vi "ICRA2024测试椭圆分裂0904有PID控制.vi"() -> ()   [LabVIEW 2018]
doc: "Demonstrates the use of the Network Streams functions to send LED status to the myRIO target."
uses:
  <vilib>/ErrorRing/Error Ring.xnode
  <vilib>/vision/NI_Vision_Development_Module.lvlib
panel:
  out "Image 8":T1(plugin-control)
  out "控制量ratio":dbl
  in  "拉伸的增益":dbl
  in  "收缩的增益":dbl
  in  "predefined control":dbl
  out "实际的ratio":dbl
  out "期望的ratio":dbl
  out "Swarm面积":sgl
  in  "期望长度":dbl
  in  "磁场开关":bool=TRUE
  out "数据总":dbl[][](array[numeric])
  out "pitch angle2":dbl[](array[numeric])
  out "pitch angle1":sgl[](array[numeric])
  out "direction angle":sgl[](array[numeric])
  out "磁场ratio":sgl[](array[numeric])
  out "磁场频率":sgl[](array[numeric])
  out "T":i32[](array[numeric])
  out "ratio":dbl[](array[numeric])
  out "长度1":i32[](array[numeric])
  out "长度2":i32[](array[numeric])
  in  "数据记录":bool
  out "长度1":i32
  out "长度2":i32
  out "Y Bottom":i32
  out "X Right":i32
  out "Y Top":i32
  out "X Left":i32
  in  "Rectangle 3":T2={"Left"=500, "Top"=800, "Right"=800, "Bottom"=1100}
  in  "Rectangle 2":T2={"Left"=500, "Top"=500, "Right"=800, "Bottom"=600}
  in  "Rectangle":T2={"Left"=500, "Top"=0, "Right"=800, "Bottom"=300}
  in  "Search Rect (entire image)":T3={"Left"=200, "Top"=120, "Right"=2000, "Bottom"=1920, "Rotation"=0.0} {"Rotation" format="%.2f"; "Left" scale=0.0..1024.0; "Right" scale=0.0..1024.0}
  out "备用的椭圆角度":sgl
  in  "Number of Erosion":i32=10
  in  "椭圆磁场开关":bool=TRUE
  out "Image 7":T1(plugin-control)
  in  "Acquisition Control::Acquisition Frame Rate":dbl=19.50304412841797 min=1.4211589097976685 max=44.94382095336914
  out "Stopped":bool
  in  "Stop (F) 2":bool caption="Stop (F)"
  out "Objects 2":T4(array[cluster]) {"Aspect Ratio" format="%.2f"; "Orientation" format="%.2f"; "Area" format="%.2f"; "Object Center"."Y" format="%.2f"; "Object Center"."X" format="%.2f"}
  in  "Settings 2":T5={"Objects"=0, "Threshold"=128, "Reject Border"=FALSE, "Fill Holes"=FALSE, "Min Object Size"=TRUE, "Min Size"=20000, "Max Object Size"=FALSE, "Max Size"=100, "Show Search Area"=FALSE, "Show Center"=TRUE, "Show Bounding Box"=TRUE} {"Objects" items=["Bright Objects", "Dark Objects"]; "Threshold" min=1 max=999999999 step=1; "Max Size" min=1 max=999999999 step=1; "Min Size" min=1 max=999999999 step=1}
  in  "Range 2":cluster{"Lower value":sgl, "Upper value":sgl}={"Lower value"=0.0, "Upper value"=230.0} {"Upper value" format="%.2f"; "Lower value" format="%.2f"}
  in  "Pause":bool
  out "Array":dbl[](array[numeric])
  in  "Parameter Settings":T6(tab)=enum."Ribbon Oscillating Field" caption="Field Types"
  in  "fg":dbl
  in  "pg":dbl
  in  "dg":dbl
  in  "Ag":dbl
  in  "AoOF":dbl
  in  "fo":sgl
  in  "do":sgl
  in  "oo":sgl
  in  "po":sgl
  in  "cc":sgl
  in  "pc":sgl
  in  "wc":sgl
  in  "dc":sgl
  in  "Ac":dbl
  in  "pr":sgl
  in  "Ar":dbl=8.0
  in  "wr":sgl=18.0
  in  "dr":sgl
  in  "Dis phase step":dbl
  in  "Dis phase frequency (Hz)":dbl
  in  "Dis tumbling frequency (Hz)":dbl
  in  "Dis strength(mT)":dbl
  in  "Swa strength (mT)":dbl
  in  "Swa frequency (Hz)":dbl
  in  "Swa pitch angle (deg)":dbl
  in  "Swa direction angle (deg)":dbl
  in  "Swa ratio":dbl=1.0
  in  "Pitch Angle (rotating around Constant, deg)":dbl
  in  "Ratio (A/C)":sgl=3.0
  in  "Direction Angle (deg)":sgl=90.0
  in  "Pitch Angle (rotating around Origin, deg)":sgl
  in  "Frequency (Hz)":sgl=6.0
  in  "Strength (mT)":dbl=3.0
  in  "Ar 2":dbl=5.0 caption="Ar"
  in  "ratio":sgl=1.0
  in  "运动方向":sgl
  in  "长轴方向":sgl
  in  "wr  2":sgl=8.0
  in  "速度大小":sgl
  out "时间":i32
  out "Numeric 5":i32
  in  "Stop":bool
  out "error out":errorcluster
  in  "Target IP Address":string="172.22.11.2"
  # "Overview: Magnetic field calculation, and send parameters to myRIO\nInstructions:\n1. Verify the value of Target IP Address. Set Visa resource name.\n2. Ensure RT Main.vi is already running. \n3. Run this VI. Set parameters of magnetic field."
  # "Strength (mT)"
  # "Pitch Angle (deg)"
  # "Direction Angle (deg)"
  # "Frequency (Hz)"
  # "Strength (mT)"
  # "Oscilation Frequency (Hz)"
  # "Oscilation Angle (deg)"
  # "Pitch Angle (deg)"
  # "Direction Angle (deg)"
  # "Strength (mT)"
  # "Frequency (Hz)"
  # "Pitch Angle (deg)"
  # "Direction Angle (deg)"
  # "Conical Angle (deg)"
  # "Strength (mT)"
  # "Frequency (Hz)"
  # "Pitch Angle (deg)"
  # "Direction Angle (deg)"
  # "Strength (mT)"
  # "Tumbling Frequency (Hz)"
  # "Phase Frequency (Hz)"
  # "Phase Step"
  # "Strength (mT)"
  # "Frequency (Hz)"
  # "Pitch Angle (deg)"
  # "Direction Angle (deg)"
  # "Ratio"
  # "Strength (mT)"
  # "Frequency (Hz)"
  # "Ratio (A/C)"
  # "Direction Angle (deg)"
  # "Pitch Angle (rotating around Origin, deg)"
  # "Pitch Angle (rotating around Constant, deg)"
  # "Strength (mT)"
  # "Frequency (Hz)"
  # "Pitch Angle  (deg)"
  # "longaxis"
  # "Direction Angle (deg)"
  # "ratio (l/s)"
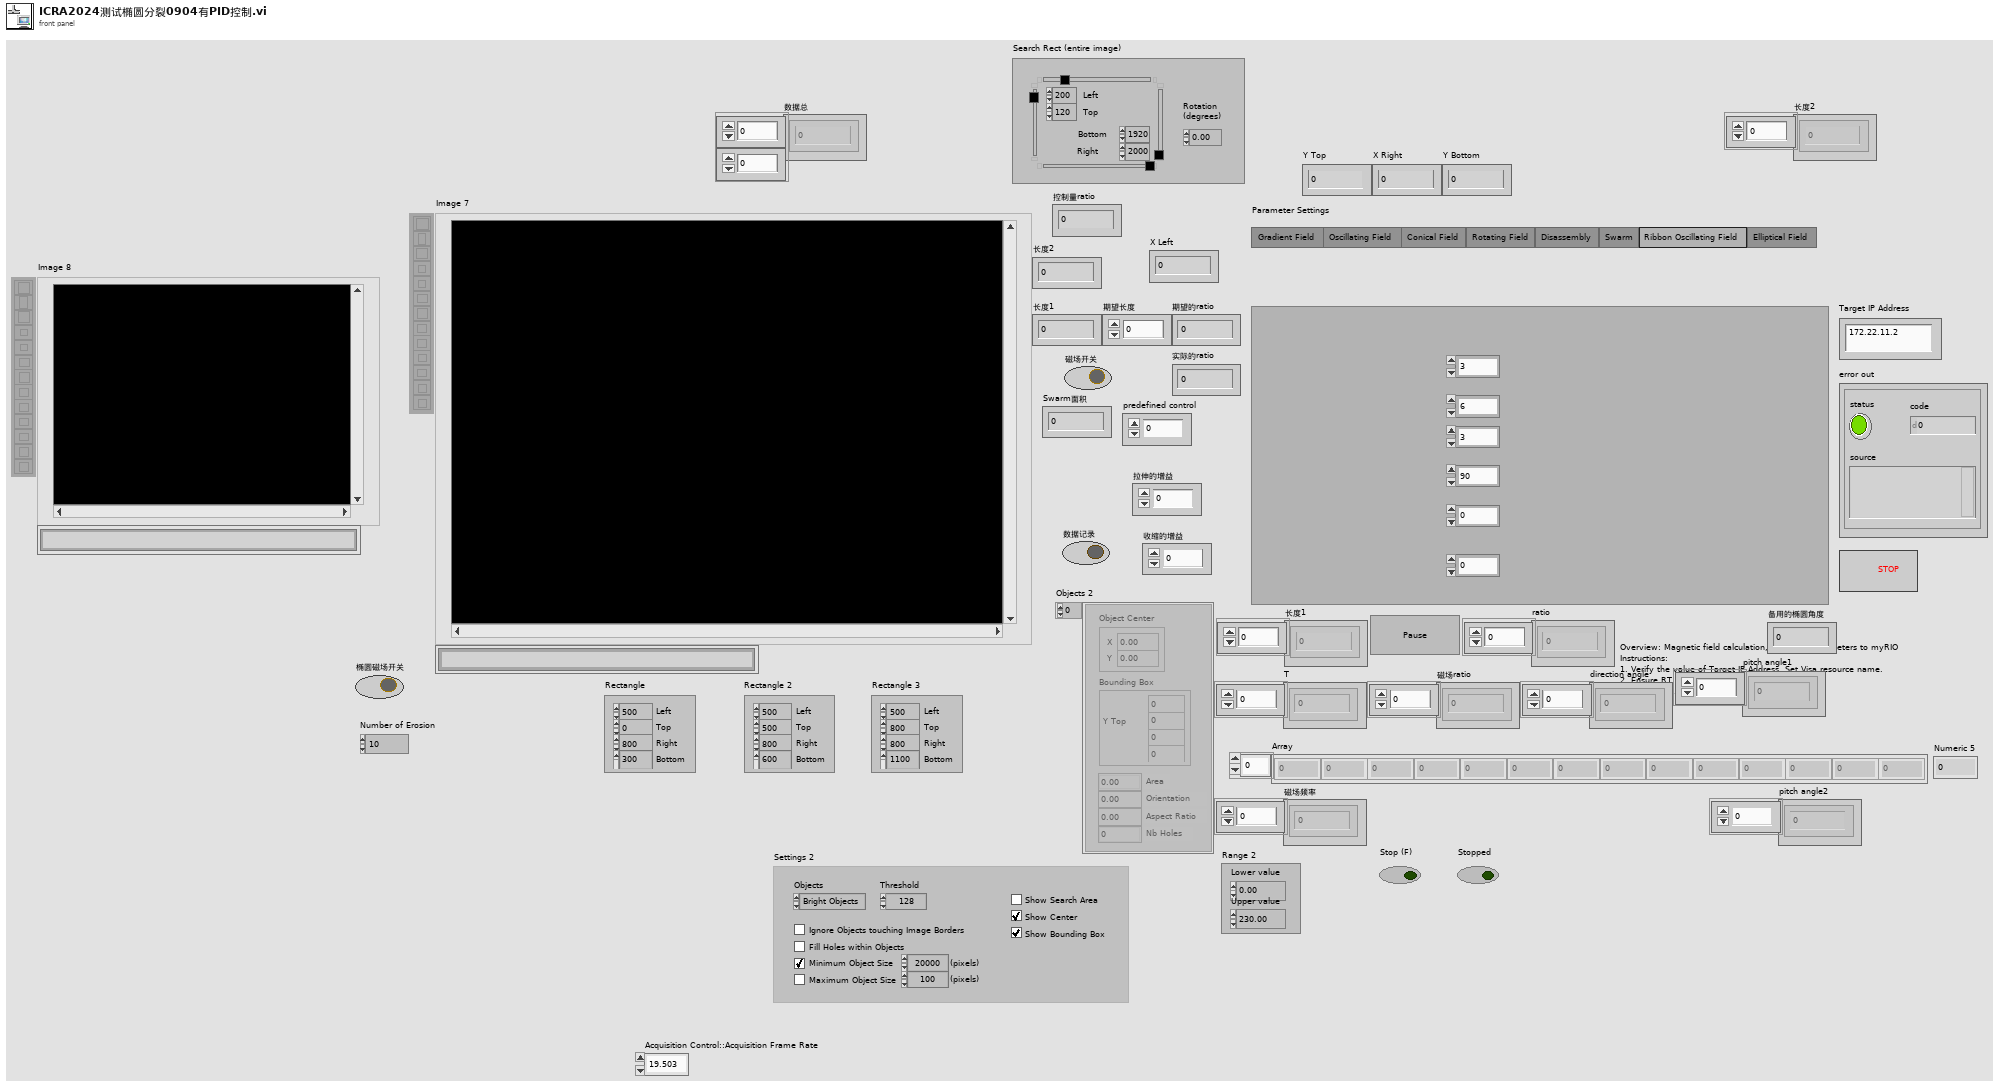
[diagram p1: front panel]
types:
  T1 = typedef "IMAQ Image.ctl" = refnum<image>
  T2 = cluster{"Left":i32, "Top":i32, "Right":i32, "Bottom":i32}
  T3 = typedef "IMAQ Rectangle" = cluster{"Left":i32, "Top":i32, "Right":i32, "Bottom":i32, "Rotation":dbl}
  T4 = cluster{"Object Center":cluster{"X":sgl, "Y":sgl}, "Bounding Box":cluster{"X Left":i32, "Y Top":i32, "X Right":i32, "Y Bottom":i32}, "Area":sgl, "Orientation":sgl, "Aspect Ratio":sgl, "Nb Holes":i32}[]
  T5 = cluster{"Objects":u16, "Threshold":i32, "Reject Border":bool, "Fill Holes":bool, "Min Object Size":bool, "Min Size":i32, "Max Object Size":bool, "Max Size":i32, "Show Search Area":bool, "Show Center":bool, "Show Bounding Box":bool}
  T6 = enum32{"Gradient Field ", "Oscillating Field", "Conical Field", "Rotating Field", "Disassembly", "Swarm", "Ribbon Oscillating Field", "Elliptical Field"}
  T7 = enum32{"AutoM", "Close", "Dilate", "Erode", "Gradient", "Gradient in", "Gradient out", "HitMiss", "Open", "PClose", "POpen", "Thick", "Thin"}
  T8 = typedef "Image Type" = u32
  T9 = cluster{"Objects[0]":cluster{"Object Center":cluster{"X":sgl, "Y":sgl}, "Bounding Box":cluster{"X Left":i32, "Y Top":i32, "X Right":i32, "Y Bottom":i32}, "Area":sgl, "Orientation":sgl, "Aspect Ratio":sgl, "Nb Holes":i32}, "Objects[1]":cluster{"Object Center":cluster{"X":sgl, "Y":sgl}, "Bounding Box":cluster{"X Left":i32, "Y Top":i32, "X Right":i32, "Y Bottom":i32}, "Area":sgl, "Orientation":sgl, "Aspect Ratio":sgl, "Nb Holes":i32}, "Objects[2]":cluster{"Object Center":cluster{"X":sgl, "Y":sgl}, "Bounding Box":cluster{"X Left":i32, "Y Top":i32, "X Right":i32, "Y Bottom":i32}, "Area":sgl, "Orientation":sgl, "Aspect Ratio":sgl, "Nb Holes":i32}, "Objects[3]":cluster{"Object Center":cluster{"X":sgl, "Y":sgl}, "Bounding Box":cluster{"X Left":i32, "Y Top":i32, "X Right":i32, "Y Bottom":i32}, "Area":sgl, "Orientation":sgl, "Aspect Ratio":sgl, "Nb Holes":i32}, "Objects[4]":cluster{"Object Center":cluster{"X":sgl, "Y":sgl}, "Bounding Box":cluster{"X Left":i32, "Y Top":i32, "X Right":i32, "Y Bottom":i32}, "Area":sgl, "Orientation":sgl, "Aspect Ratio":sgl, "Nb Holes":i32}, "Objects[5]":cluster{"Object Center":cluster{"X":sgl, "Y":sgl}, "Bounding Box":cluster{"X Left":i32, "Y Top":i32, "X Right":i32, "Y Bottom":i32}, "Area":sgl, "Orientation":sgl, "Aspect Ratio":sgl, "Nb Holes":i32}, "Objects[6]":cluster{"Object Center":cluster{"X":sgl, "Y":sgl}, "Bounding Box":cluster{"X Left":i32, "Y Top":i32, "X Right":i32, "Y Bottom":i32}, "Area":sgl, "Orientation":sgl, "Aspect Ratio":sgl, "Nb Holes":i32}, "Objects[7]":cluster{"Object Center":cluster{"X":sgl, "Y":sgl}, "Bounding Box":cluster{"X Left":i32, "Y Top":i32, "X Right":i32, "Y Bottom":i32}, "Area":sgl, "Orientation":sgl, "Aspect Ratio":sgl, "Nb Holes":i32}, "Objects[8]":cluster{"Object Center":cluster{"X":sgl, "Y":sgl}, "Bounding Box":cluster{"X Left":i32, "Y Top":i32, "X Right":i32, "Y Bottom":i32}, "Area":sgl, "Orientation":sgl, "Aspect Ratio":sgl, "Nb Holes":i32}}
  T10 = cluster{"Object Center":cluster{"X":sgl, "Y":sgl}, "Bounding Box":cluster{"X Left":i32, "Y Top":i32, "X Right":i32, "Y Bottom":i32}, "Area":sgl, "Orientation":sgl, "Aspect Ratio":sgl, "Nb Holes":i32}
  T11 = cluster{"X Left":i32, "Y Top":i32, "X Right":i32, "Y Bottom":i32}
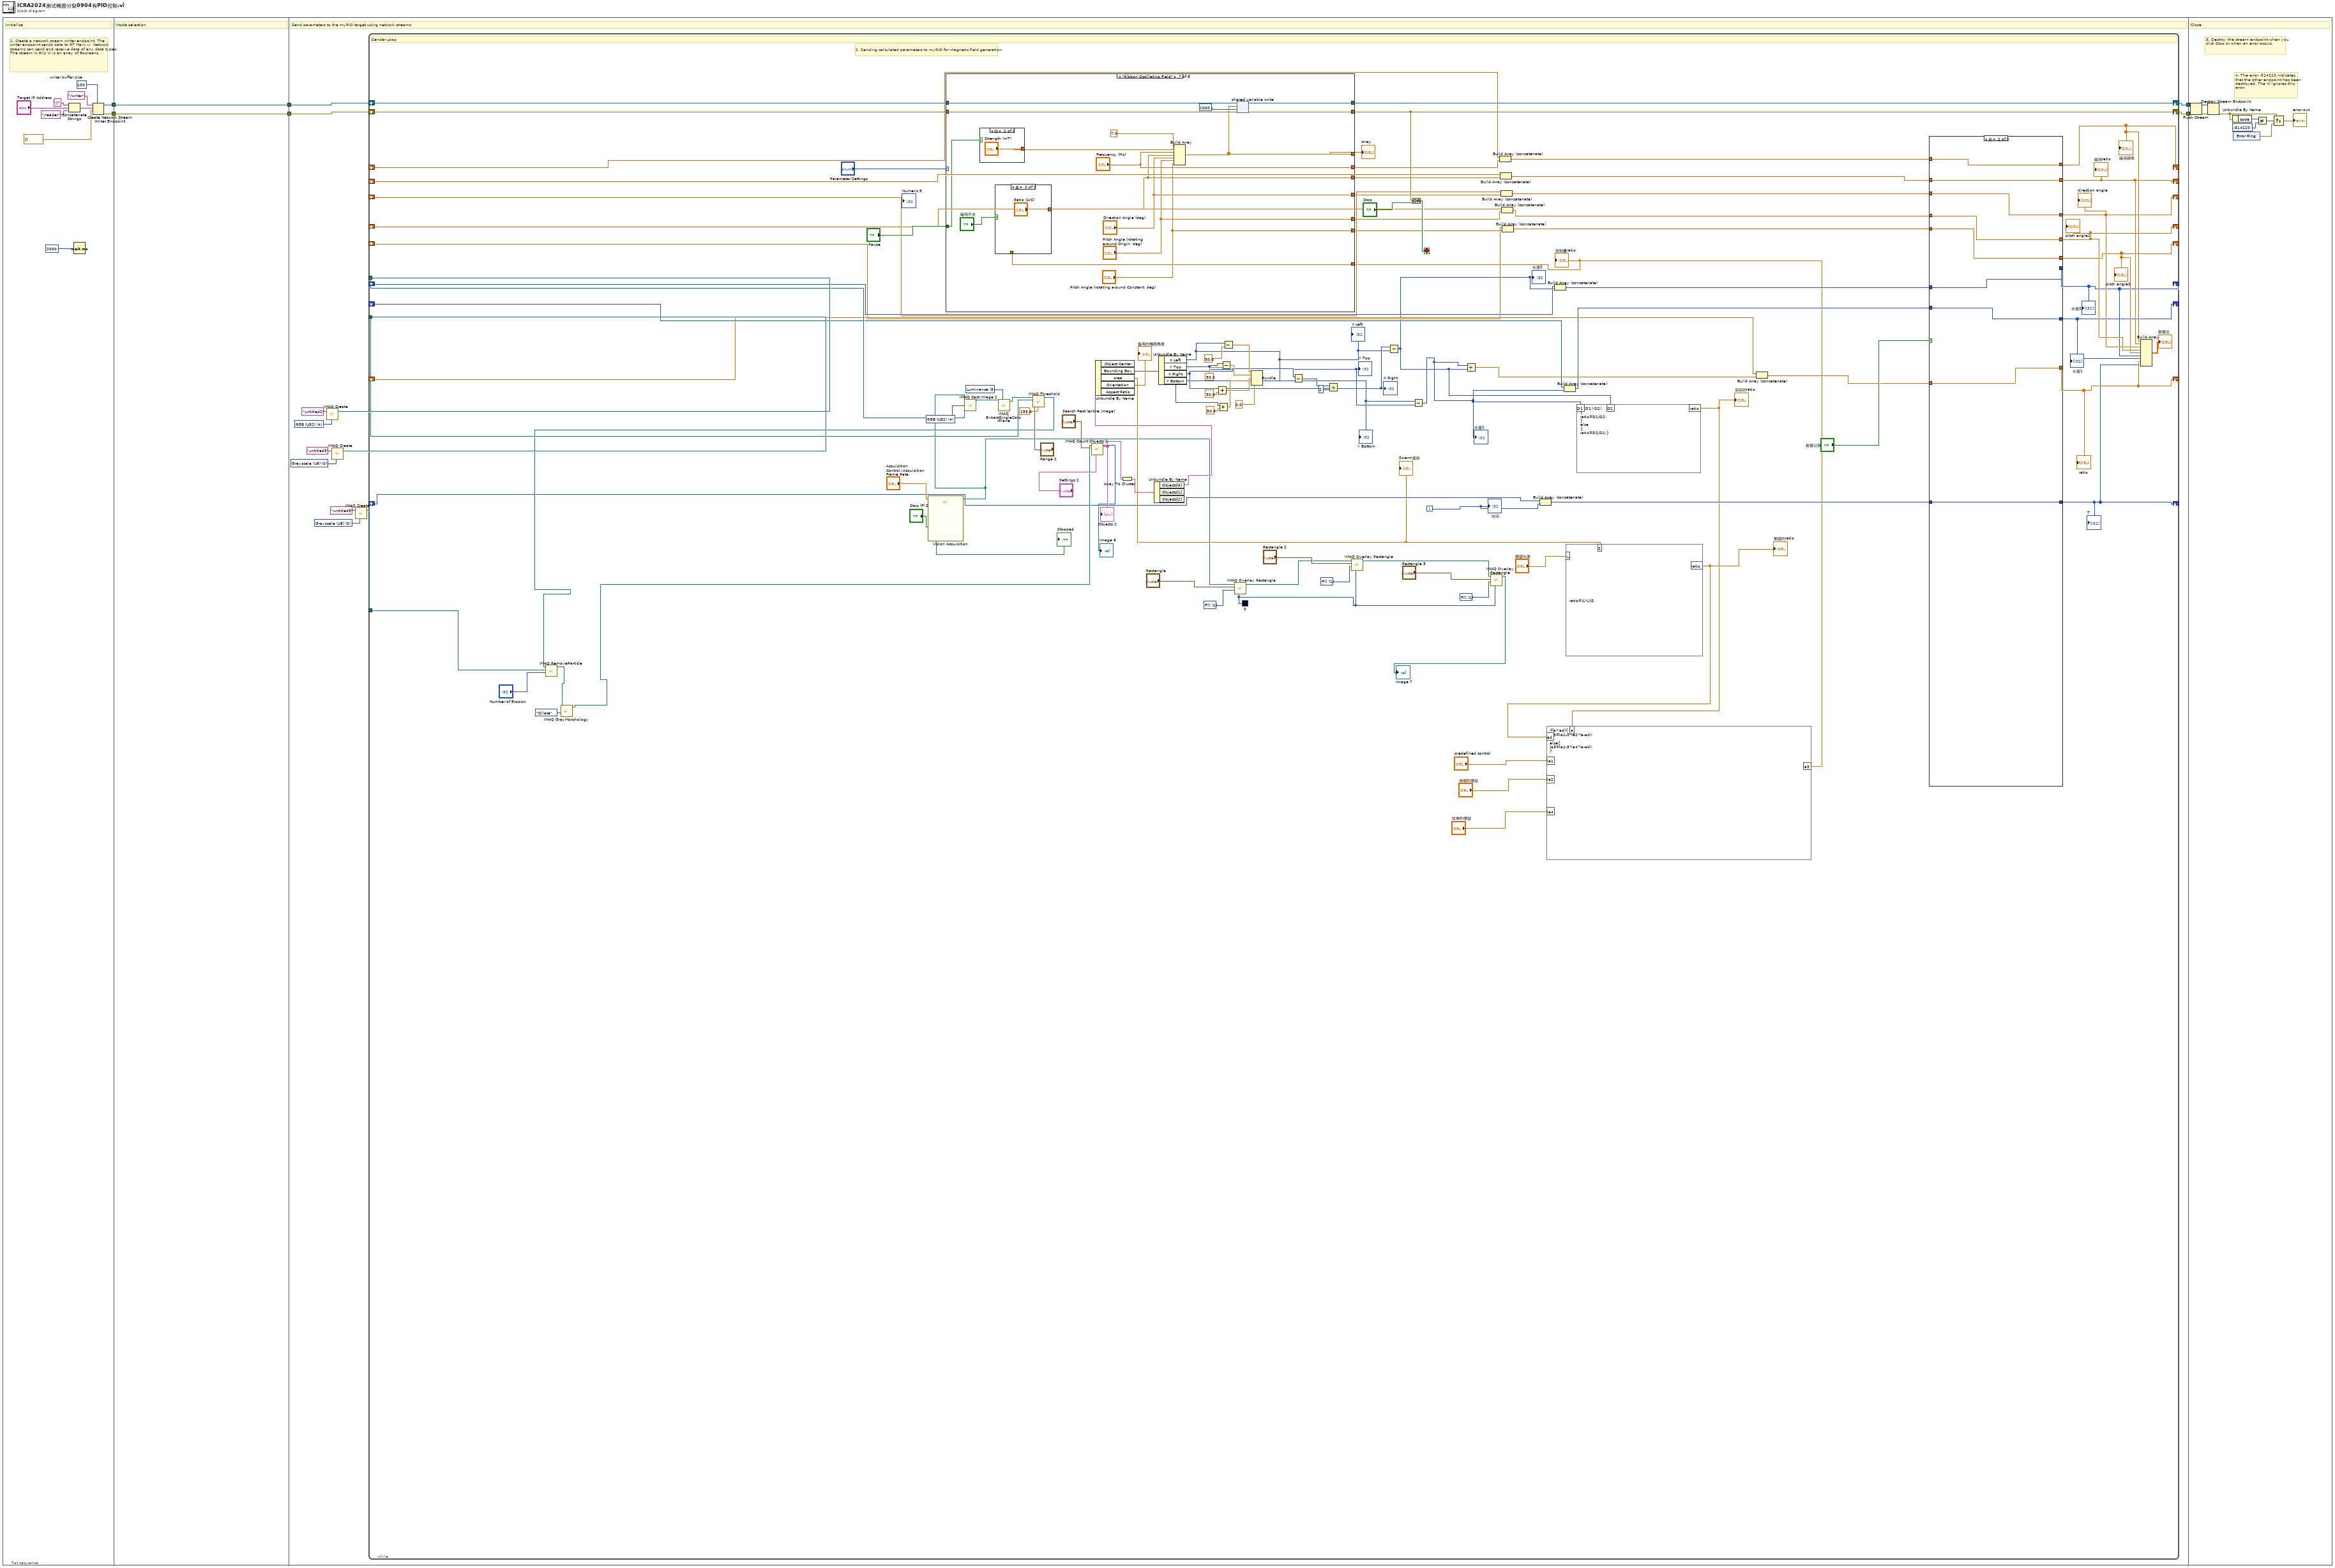
[diagram p0: block diagram]
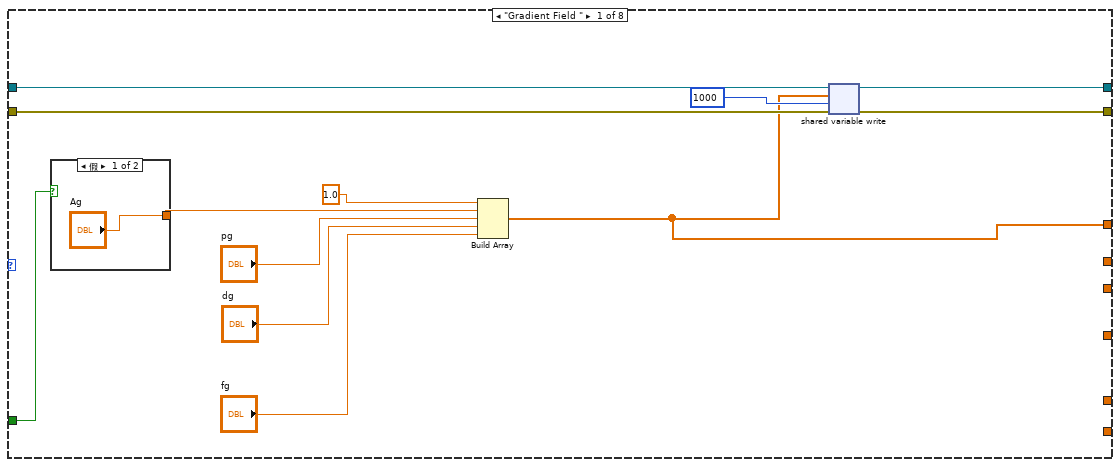
[diagram p3: hidden frame]
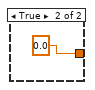
[diagram p4: hidden frame]
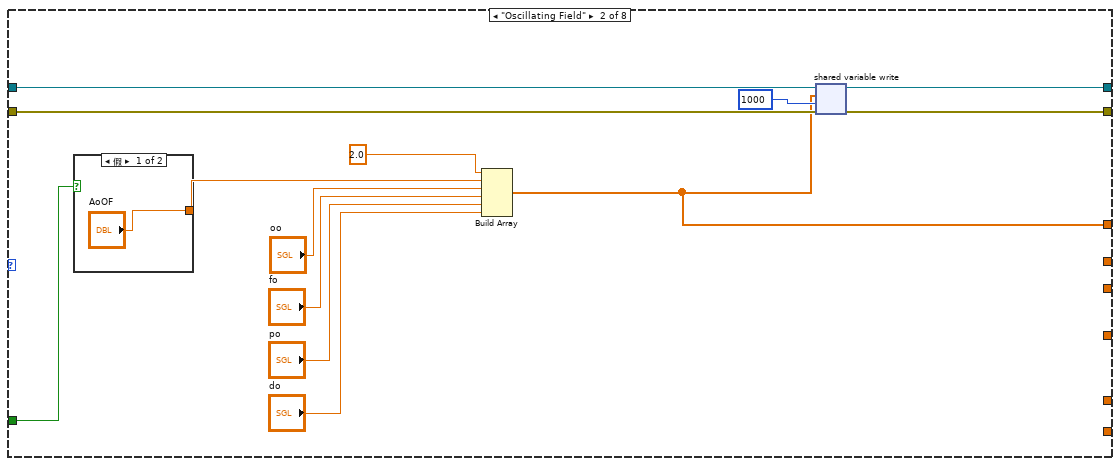
[diagram p5: hidden frame]
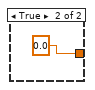
[diagram p6: hidden frame]
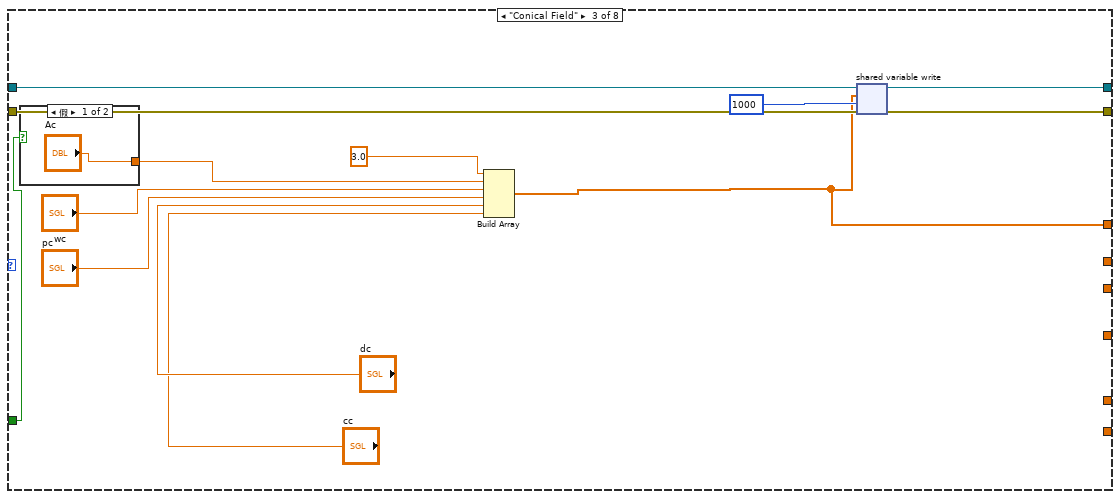
[diagram p7: hidden frame]
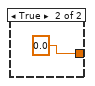
[diagram p8: hidden frame]
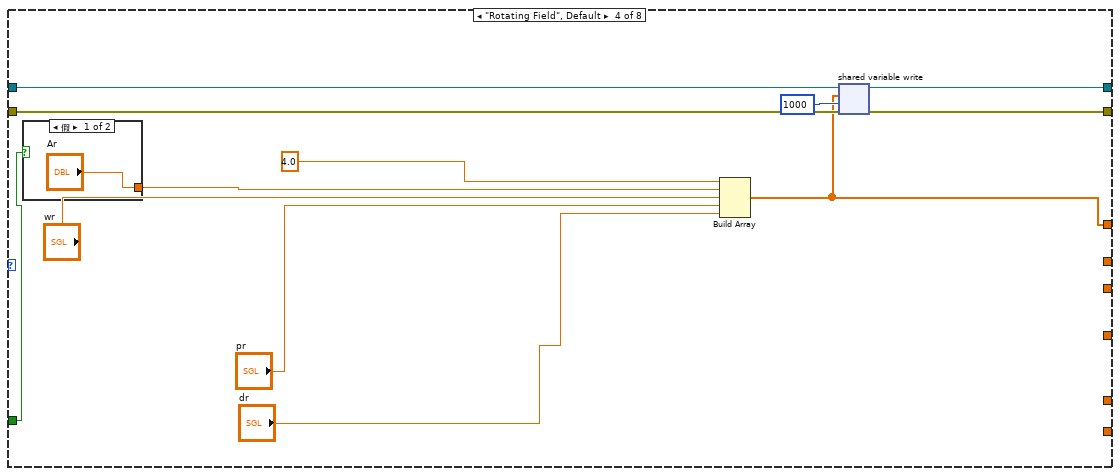
[diagram p9: hidden frame]
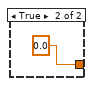
[diagram p10: hidden frame]
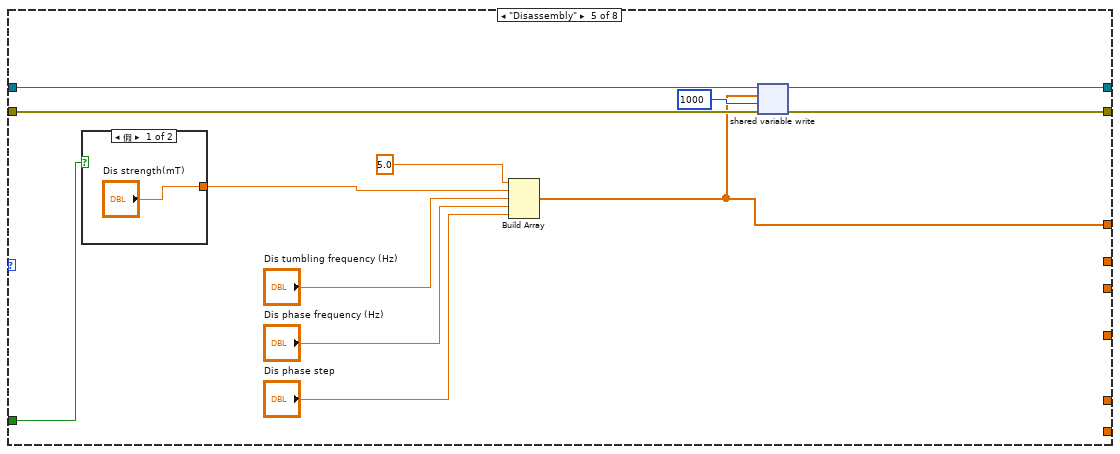
[diagram p11: hidden frame]
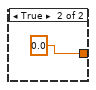
[diagram p12: hidden frame]
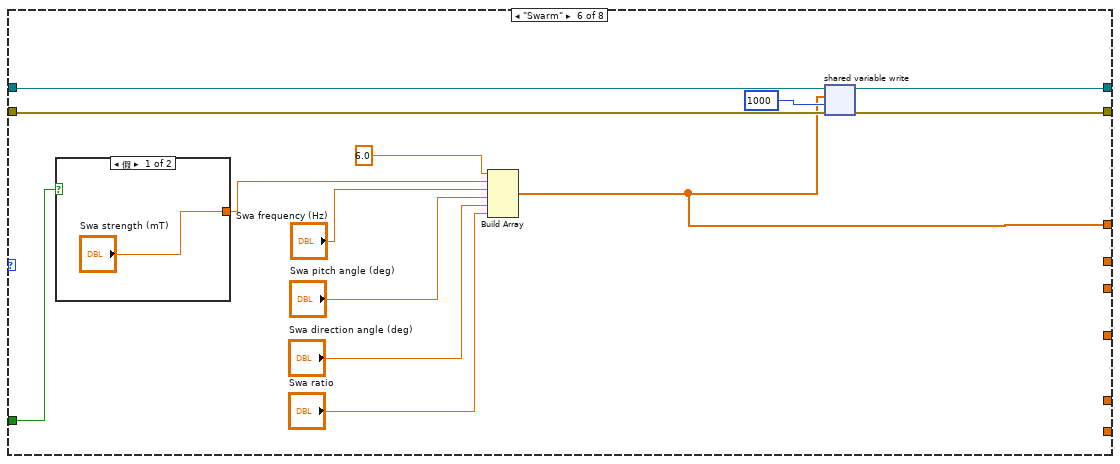
[diagram p13: hidden frame]
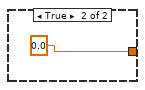
[diagram p14: hidden frame]
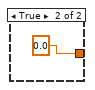
[diagram p16: hidden frame]
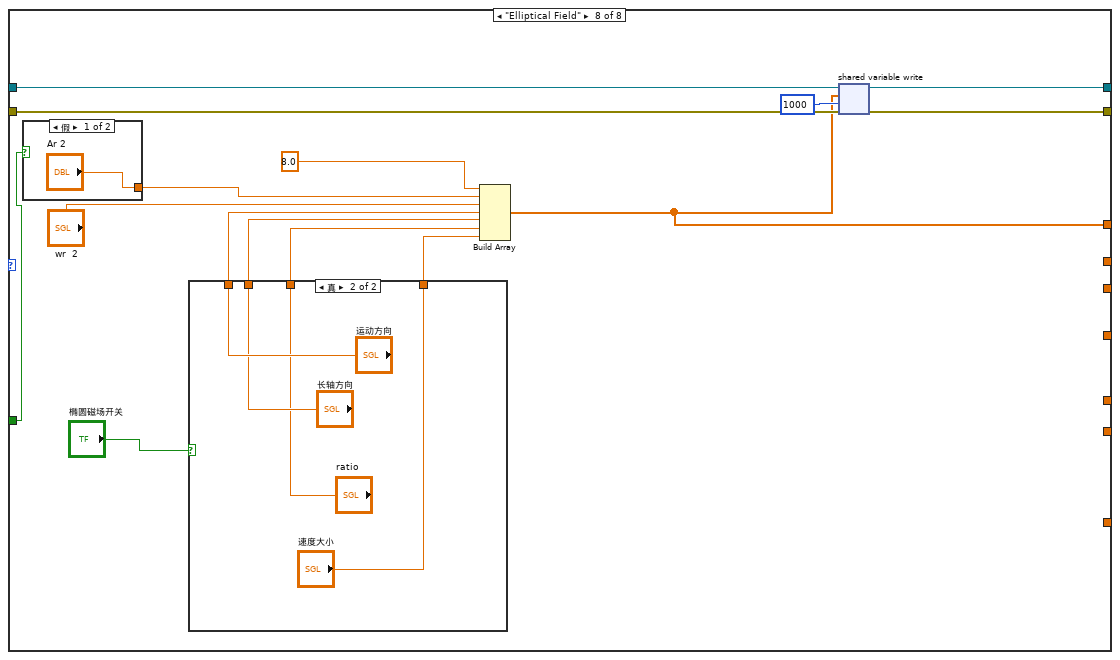
[diagram p17: hidden frame]
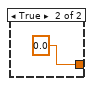
[diagram p19: hidden frame]
diagram:
  n1 = flat-sequence {
    tunnel: [w11] -> w2
    tunnel: [w10] -> w1
    tunnel: [w18] -> w4
    tunnel: [w17] -> w3
    tunnel: w1 -> [w17]
    tunnel: w2 -> [w18]
    tunnel: [w29] -> w6
    tunnel: w4 -> [w31]
    tunnel: [w28] -> w5
    tunnel: w3 -> [w30]
    tunnel: w6 -> [w284]
    tunnel: w5 -> [w281]
    frame #0 {
      w9 = 100  # writer buffer size
      # "1. Create a network stream writer endpoint. The writer endpoint sends data to RT Main.vi. Network streams can send and receive data of any data types. The stream in this VI is an array of Booleans."
      # "Initialize"
      n2 = Concatenate Strings("//", "Target IP Address", "/reader") -> (w16:string)
      n3 = Wait (ms)(milliseconds to wait=2000) -> ()  [unwired: 1 out]
      n4 = Create Network Stream Writer Endpoint(7:w9, 9:dbl[] [], 10:w16, 11:"/writer" ("reader name")) -> (0:w10:errorcluster, 3:w11:refnum<k21>)  [unwired: 3 in]
    }
    frame #1 {
      # "Mode selection"
    }
    frame #2 {
      w20 = T8 0 items=["Grayscale (U8)", "Grayscale (I16)", "Grayscale (SGL)", "Complex (CSG)", "RGB (U32)", "HSL (U32)", "RGB (U64)", "Grayscale (U16)"] ("Image Type")
      w24 = T8 0 items=["Grayscale (U8)", "Grayscale (I16)", "Grayscale (SGL)", "Complex (CSG)", "RGB (U32)", "HSL (U32)", "RGB (U64)", "Grayscale (U16)"] ("Image Type")
      w26 = T8 4 items=["Grayscale (U8)", "Grayscale (I16)", "Grayscale (SGL)", "Complex (CSG)", "RGB (U32)", "HSL (U32)", "RGB (U64)", "Grayscale (U16)"] ("Image Type")
      # "Send parameters to the myRIO target using network streams"
      n5 = call "IMAQ Create"("Image Name"="untitled2", "Image Type"=w26) -> ("New Image"=w23:T1)  [unwired: 3 in, 1 out]
      n6 = call "IMAQ Create"("Image Name"="untitled3", "Image Type"=w24) -> ("New Image"=w22:T1)  [unwired: 3 in, 1 out]
      n7 = call "IMAQ Create"("Image Name"="untitled3", "Image Type"=w20) -> ("New Image"=w19:T1)  [unwired: 3 in, 1 out]
      n8 = while {
        shift-right: [w133] -> w28
        shift-left: w30 -> [w135]
        shift-right: [w134] -> w29
        shift-left: w31 -> [w136]
        tunnel: w22 -> [w124]
        tunnel: w23 -> [w119]
        tunnel: w19 -> [w104]
        shift-right: [w48] -> _
        shift-left: _ -> [w77]
        shift-right: [w47] -> _
        shift-left: _ -> [w75]
        shift-right: [w46] -> _
        shift-left: _ -> [w72]
        shift-right: [w45] -> _
        shift-left: _ -> [w69]
        shift-right: [w53] -> _
        shift-left: _ -> [w66]
        shift-right: [w52] -> _
        shift-left: _ -> [w63]
        shift-right: [w51] -> _
        shift-left: _ -> [w60]
        shift-right: [w50] -> _
        shift-left: _ -> [w57]
        shift-right: [w49] -> _
        shift-left: _ -> [w54]
        i -> [w71]
        stop <- w123 stop-if-true
        w84 = u32 0 ("Color")
        w87 = u32 1 items=["Frame", "Fill", "Highlight"] ("Drawing Mode (Frame)")
        w89 = u32 1 items=["Frame", "Fill", "Highlight"] ("Drawing Mode (Frame)")
        w93 = u32 1 items=["Frame", "Fill", "Highlight"] ("Drawing Mode (Frame)")
        w118 = T8 4 items=["Grayscale (U8)", "Grayscale (I16)", "Grayscale (SGL)", "Complex (CSG)", "RGB (U32)", "HSL (U32)", "RGB (U64)", "Grayscale (U16)"] ("Image Type")
        w129 = 5 items=["Red", "Green", "Blue", "Hue", "Saturation", "Luminance", "Value", "Intensity"] ("Color Plane")
        # "2. Sending calculated parameters to myRIO for magnetic field generation."
        # "Sender Loop"
        n9 = call "Vision Acquisition"("Acquisition Control::Acquisition Frame Rate"="Acquisition Control::Acquisition Frame Rate", "Stop (F)"="Stop (F) 2") -> ("Image Out"=w33:T1, "Stopped"=→"Stopped":bool)  [unwired: 23 in, 1 out]
        n10 = call "IMAQ Cast Image 2"("Image Src"=w33, "Image Dst"=w119, "Image Type"=w118) -> ("Image Dst Out"=w120:T1)  [unwired: 11 in, 1 out]
        n11 = call "IMAQ ExtractSingleColorPlane"("Color Plane"=w129, "Image Src"=w120) -> ("Image Dst Out"=w99:T1)  [unwired: 8 in, 1 out]
        n12 = call "IMAQ Threshold"("Replace Value"=sgl 255.0, "Range"="Range 2", "Image Dst"=w124, "Image Src"=w99) -> ("Image Dst Out"=w105:T1)  [unwired: 6 in, 1 out]
        n13 = call "IMAQ RemoveParticle"("Number of Erosion"="Number of Erosion", "Image Dst"=w104, "Image Src"=w105) -> ("Image Dst Out"=w102:T1)  [unwired: 7 in, 1 out]
        n14 = call "IMAQ GrayMorphology"("Operation"=T7."Dilate", "Image Src"=w102) -> ("Image Dst Out"=w100:T1)  [unwired: 8 in, 1 out]
        n15 = call "IMAQ Count Objects 2"("Settings"="Settings 2", "Search Rect (entire image)"="Search Rect (entire image)", "Image"=w100) -> ("Image Out"=→"Image 8":T1, "Objects"=w125:T4)  [unwired: 4 in, 3 out]
        "Objects 2" <- w125
        n16 = Array To Cluster(array=w125) -> (cluster=w107:T9)
        n17 = Unbundle By Name(w107) -> ("Objects[0]"=w106:T10)  [unwired: 2 out]
        n18 = Unbundle By Name(w106) -> ("Bounding Box"=w117:T11, "Area"=w42:sgl, "Orientation"=→"备用的椭圆角度":sgl)  [unwired: 2 out]
        "Swarm面积" <- w42
        n19 = Unbundle By Name(w117) -> ("X Left"=w82:i32, "Y Top"=w80:i32, "X Right"=w83:i32, "Y Bottom"=w81:i32)
        "X Left" <- w82
        "Y Top" <- w80
        "X Right" <- w83
        "Y Bottom" <- w81
        n20 = Add(x=w83, y=50.0) -> (x+y=w110:dbl)
        n21 = Add(x=w81, y=50.0) -> (x+y=w109:dbl)
        n22 = Subtract(x=w80, y=50.0) -> (x-y=w111:dbl)
        n23 = Subtract(x=w82, y=50.0) -> (x-y=w112:dbl)
        n24 = call "IMAQ Overlay Rectangle"("Color"=w84, "Drawing Mode (Frame)"=w93, "Rectangle"="Rectangle", "Image"=w33) -> ("Image Out"=w90:T1)  [unwired: 6 in, 1 out]
        n25 = Bundle(w112, w111, w110, w109, 0.0) -> ()  [unwired: 1 in, 1 out]
        n26 = Subtract(x=w83, y=w82) -> (x-y=w96:i32)
        n27 = Divide(x=w96, y=2) -> ()  [unwired: 1 out]
        n28 = call "IMAQ Overlay Rectangle"("Color"=w84, "Drawing Mode (Frame)"=w89, "Rectangle"="Rectangle 2", "Image"=w90) -> ("Image Out"=w86:T1)  [unwired: 6 in, 1 out]
        n29 = Subtract(x=w83, y=w82) -> (x-y=w39:i32)
        "长度2" <- w39
        n30 = Subtract(x=w81, y=w80) -> (x-y=w40:i32)
        "长度1" <- w40
        n31 = Divide(x=w40, y=w39) -> (x/y=w74:dbl)
        n32 = call "IMAQ Overlay Rectangle"("Color"=w84, "Drawing Mode (Frame)"=w87, "Rectangle"="Rectangle 3", "Image"=w86) -> ("Image Out"=→"Image 7":T1)  [unwired: 6 in, 1 out]
        n33 = Build Array (concatenate)(w69, w71) -> (w70:i32[])
        n34 = Build Array (concatenate)(w77, w39) -> (w78:i32[])
        n35 = Build Array (concatenate)(w75, w40) -> (w76:i32[])
        n36 = formula code="ratio=(L*L)/S;"("L"="期望长度", "S"=w42) -> ("ratio"=w41:dbl)
        "期望的ratio" <- w41
        n37 = formula code="if (D1>D2)\n{\nratio=D1/D2;\n}\nelse\n{\nratio=D2/D1;}"("D1"=w40, "D2"=w39) -> ("ratio"=w38:dbl)
        "实际的ratio" <- w38
        n38 = formula code="if(a>ad){\nla3=la1-3*la2*(a-ad);\n}\nelse{\nla3=la1-3*la4*(a-ad);\n}"("ad"=w41, "a"=w38, "la1"="predefined control", "la2"="收缩的增益", "la4"="拉伸的增益") -> ("la3"=w34:dbl)
        "控制量ratio" <- w34
        n39 = case shown="\"Ribbon Oscillating Field\"" "Parameter Settings" {
          tunnel: w136 -> [w157 w172 w187 w201 w215 w229 w249 w267]
          tunnel: w135 -> [w154 w171 w186 w200 w213 w228 w247 w266]
          tunnel: [w156 w170 w184 w199 w214 w227 w248 w265] -> w134
          tunnel: [w155 w169 w185 w198 w212 w226 w246 w264] -> w133
          tunnel: [w150 w163 w178 w193 w206 w221 w244 w259] -> w132
          tunnel: "Pause" -> [w148 w161 w176 w191 w205 w220 w242 w257]
          tunnel: [_ _ _ _ _ _ "Frequency (Hz)" _] -> w68
          tunnel: [_ _ _ _ _ _ w239 _] -> w65
          tunnel: [_ _ _ _ _ _ "Direction Angle (deg)" _] -> w62
          tunnel: [_ _ _ _ _ _ "Pitch Angle (rotating around Origin, deg)" _] -> w59
          tunnel: [_ _ _ _ _ _ "Pitch Angle (rotating around Constant, deg)" _] -> w56
          tunnel: w34 -> [_ _ _ _ _ _ w234 _]
          frame "Gradient Field " {
            n40 = case shown="假" w148 {
              tunnel: ["Ag" 0.0] -> w149
              frame False {
              }
              frame True {
              }
            }
            n41 = Build Array(1.0, w149, "pg", "dg", "fg") -> (w150:dbl[])
            n42 = shared-variable-write(w157, w154, w150, 1000 ("timeout ms (-1)")) -> (w156:refnum<k21>, w155:errorcluster)  [unwired: 1 out]
          }
          frame "Oscillating Field" {
            n43 = case shown="假" w161 {
              tunnel: ["AoOF" 0.0] -> w162
              frame False {
              }
              frame True {
              }
            }
            n44 = Build Array(2.0, w162, "oo", "fo", "po", "do") -> (w163:dbl[])
            n45 = shared-variable-write(w172, w171, w163, 1000 ("timeout ms (-1)")) -> (w170:refnum<k21>, w169:errorcluster)  [unwired: 1 out]
          }
          frame "Conical Field" {
            # "FG"
            n46 = case shown="假" w176 {
              tunnel: ["Ac" 0.0] -> w177
              frame False {
              }
              frame True {
              }
            }
            n47 = Build Array(3.0, w177, "wc", "pc", "dc", "cc") -> (w178:dbl[])
            n48 = shared-variable-write(w187, w186, w178, 1000 ("timeout ms (-1)")) -> (w184:refnum<k21>, w185:errorcluster)  [unwired: 1 out]
          }
          frame "Rotating Field", Default {
            n49 = case shown="假" w191 {
              tunnel: ["Ar" 0.0] -> w192
              frame False {
              }
              frame True {
              }
            }
            n50 = Build Array(4.0, w192, "wr", "pr", "dr") -> (w193:dbl[])
            n51 = shared-variable-write(w201, w200, w193, 1000 ("timeout ms (-1)")) -> (w199:refnum<k21>, w198:errorcluster)  [unwired: 1 out]
          }
          frame "Disassembly" {
            n52 = case shown="假" w205 {
              tunnel: ["Dis strength(mT)" 0.0] -> w210
              frame False {
              }
              frame True {
              }
            }
            n53 = Build Array(5.0, w210, "Dis tumbling frequency (Hz)", "Dis phase frequency (Hz)", "Dis phase step") -> (w206:dbl[])
            n54 = shared-variable-write(w215, w213, w206, 1000 ("timeout ms (-1)")) -> (w214:refnum<k21>, w212:errorcluster)  [unwired: 1 out]
          }
          frame "Swarm" {
            n55 = case shown="假" w220 {
              tunnel: ["Swa strength (mT)" 0.0] -> w219
              frame False {
              }
              frame True {
              }
            }
            n56 = Build Array(6.0, w219, "Swa frequency (Hz)", "Swa pitch angle (deg)", "Swa direction angle (deg)", "Swa ratio") -> (w221:dbl[])
            n57 = shared-variable-write(w229, w228, w221, 1000 ("timeout ms (-1)")) -> (w227:refnum<k21>, w226:errorcluster)  [unwired: 1 out]
          }
          frame "Ribbon Oscillating Field" {
            n58 = case shown="假" w242 {
              tunnel: ["Strength (mT)" 0.0] -> w241
              frame False {
              }
              frame True {
              }
            }
            n59 = case shown="真" "磁场开关" {
              tunnel: [w250 "Ratio (A/C)"] -> w239
              tunnel: w234 -> [w250 _]
              frame False {
              }
              frame True {
              }
            }
            n60 = Build Array(7.0, w241, "Frequency (Hz)", w239, "Direction Angle (deg)", "Pitch Angle (rotating around Origin, deg)", "Pitch Angle (rotating around Constant, deg)") -> (w244:dbl[])
            n61 = shared-variable-write(w249, w247, w244, 1000 ("timeout ms (-1)")) -> (w248:refnum<k21>, w246:errorcluster)  [unwired: 1 out]
          }
          frame "Elliptical Field" {
            n62 = case shown="假" w257 {
              tunnel: ["Ar 2" 0.0] -> w258
              frame False {
              }
              frame True {
              }
            }
            n63 = case shown="真" "椭圆磁场开关" {
              tunnel: [_ "运动方向"] -> w262
              tunnel: [_ "长轴方向"] -> w261
              tunnel: [_ "ratio"] -> w256
              tunnel: [_ "速度大小"] -> w255
              frame False {
              }
              frame True {
              }
            }
            n64 = Build Array(8.0, w258, "wr  2", w262, w261, w256, w255) -> (w259:dbl[])
            n65 = shared-variable-write(w267, w266, w259, 1000 ("timeout ms (-1)")) -> (w265:refnum<k21>, w264:errorcluster)  [unwired: 1 out]
          }
        }
        "Array" <- w132
        n66 = Or(x=w133, y="Stop") -> (x .or. y?=w123:bool)
        n67 = Build Array (concatenate)(w66, w68) -> (w67:sgl[])
        n68 = Build Array (concatenate)(w63, w65) -> (w64:dbl[])
        n69 = Build Array (concatenate)(w60, w62) -> (w61:sgl[])
        n70 = Build Array (concatenate)(w57, w59) -> (w58:sgl[])
        n71 = Build Array (concatenate)(w54, w56) -> (w55:dbl[])
        n72 = Build Array (concatenate)(w72, w74) -> (w73:dbl[])
        n73 = case shown="真" "数据记录" {
          tunnel: [_ w146] -> w48
          tunnel: w78 -> [_ w146]
          tunnel: [_ w145] -> w47
          tunnel: w76 -> [_ w145]
          tunnel: [_ w144] -> w46
          tunnel: w73 -> [_ w144]
          tunnel: w70 -> [_ w143]
          tunnel: [_ w143] -> w45
          tunnel: [_ w142] -> w53
          tunnel: w67 -> [_ w142]
          tunnel: [_ w141] -> w52
          tunnel: w64 -> [_ w141]
          tunnel: [_ w140] -> w51
          tunnel: w61 -> [_ w140]
          tunnel: [_ w139] -> w50
          tunnel: w58 -> [_ w139]
          tunnel: [_ w138] -> w49
          tunnel: w55 -> [_ w138]
          frame False {
          }
          frame True {
          }
        }
        "长度2" <- w48
        "长度1" <- w47
        "ratio" <- w46
        "T" <- w45
        "磁场频率" <- w53
        "磁场ratio" <- w52
        "direction angle" <- w51
        "pitch angle1" <- w50
        "pitch angle2" <- w49
        n74 = Build Array(w53, w52, w51, w50, w49, w48, w47, w46, w45) -> (→"数据总":dbl[][])
        "时间" <- w71
      }
    }
    frame #3 {
      # "4. The error -314220 indicates that the other endpoint has been destroyed. The VI ignores this error."
      # "3. Destroy the stream endpoint when you click Stop or when an error occurs."
      # "Close"
      n75 = Flush Stream(8:w281, 11:w284) -> (0:w282:errorcluster, 3:w283:refnum<k21>)  [unwired: 2 in, 1 out]
      n76 = Destroy Stream Endpoint(8:w282, 11:w283) -> (0:w276:errorcluster)
      n77 = Unbundle By Name(w276) -> ("code"=w280:i32)
      n78 = xnode "Error Ring"() -> ("错误输出"=w277:errorcluster)
      n79 = Not Equal?(x=w280, y=-314220) -> (x != y?=w278:bool)
      n80 = Select(t=w276, s=w278, f=w277) -> (s? t:f=→"error out":errorcluster)
    }
  }
